vi "test_NEO480HTA get all data.vi"(8 "Error In":errorcluster) -> (0 "Error Out":errorcluster)   [LabVIEW 2023]
uses:
  Real All CFG/Read All CFG.lvclass
  Virt Instr Host/Virt Instr Host.lvclass
  Measure and Stimulus Subsystems/Measure and Stimulus Subsystems.lvclass
panel:
  out "i":i32
  out "Absolute Humidity":dbl format="%#_g g m^-3"
  out "Pressure":dbl format="%#_g mbar"
  out "Dew Point":dbl format="%#_g °C"
  out "Temperature":dbl format="%#_g °C"
  in  "Stop":bool
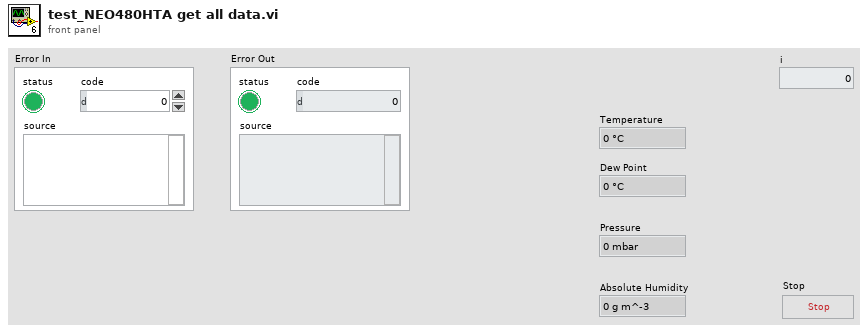
[diagram p1: front panel]
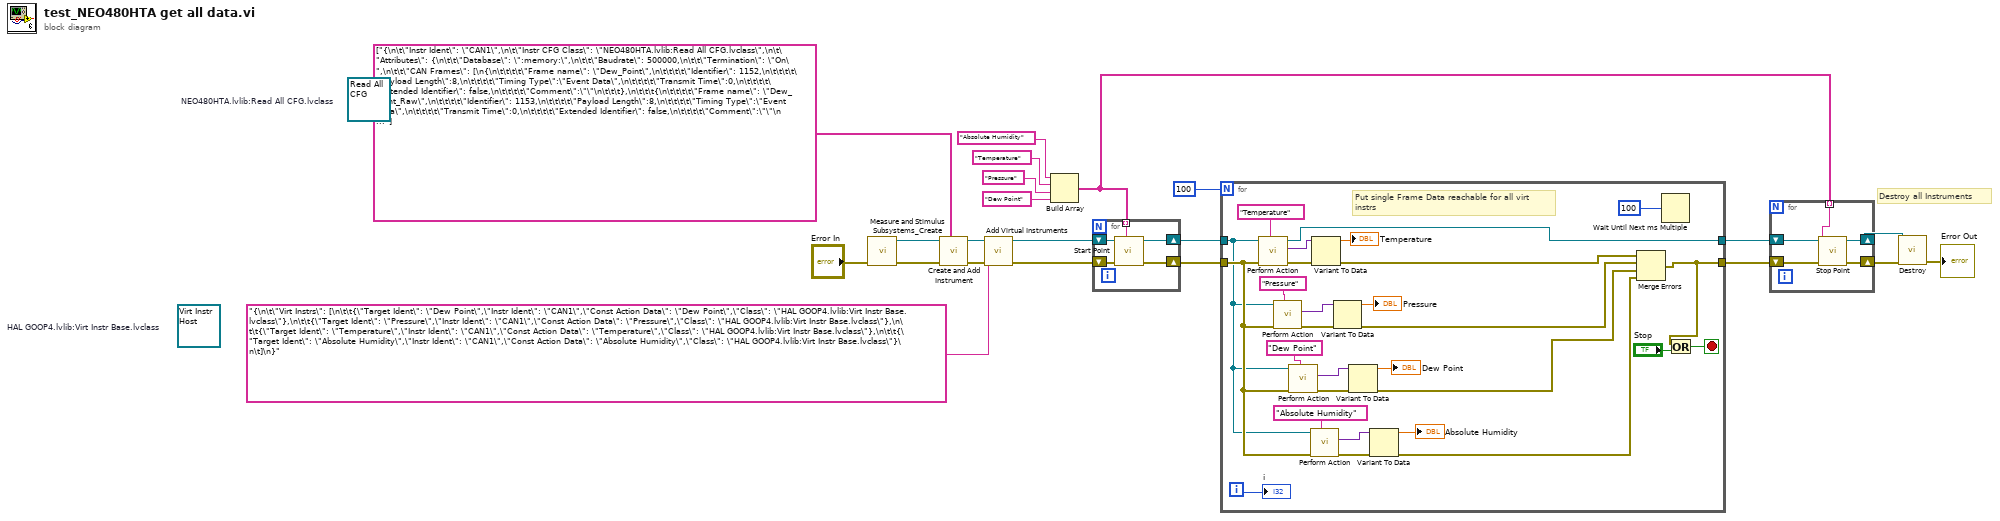
[diagram p0: block diagram]
diagram:
  (unwired) refnum<class "Virt Instr Host.lvclass"> refnum  # HAL GOOP4.lvlib:Virt Instr Base.lvclass
  (unwired) refnum<class "Read All CFG.lvclass"> refnum  # NEO480HTA.lvlib:Read All CFG.lvclass
  # "Destroy all Instruments"
  n1 = call "Measure and Stimulus Subsystems_Create.vi"("Error In"="Error In") -> ("Error Out"=w21:errorcluster, "reference out"=w22:refnum<class "Measure and Stimulus Subsystems.lvclass">)  [unwired: 9 in]
  n2 = call "Create and Add Instrument.vi"("Physical Intr Configs"=string[] ["{\n\t\"Instr Ident\": \"CAN1\",\n\t\"Instr CFG Class\": \"NEO480HTA.lvlib:Read All CFG.lvclass\",\n\t\"Attributes\": {\n\t\t\"Database\": \":memory:\",\n\t\t\"Baudrate\": 500000,\n\t\t\"Termination\": \"On\",\n\t\t\"CAN Frames\": [\n{\n\t\t\t\t\"Frame name\": \"Dew_Point\",\n\t\t\t\t\"Identifier\": 1152,\n\t\t\t\t\"Payload Length\":8,\n\t\t\t\t\"Timing Type\":\"Event Data\",\n\t\t\t\t\"Transmit Time\":0,\n\t\t\t\t\"Extended Identifier\": false,\n\t\t\t\t\"Comment\":\"\"\n\t\t\t},\n\t\t\t{\n\t\t\t\t\"Frame name\": \"Dew_Point_Raw\",\n\t\t\t\t\"Identifier\": 1153,\n\t\t\t\t\"Payload Length\":8,\n\t\t\t\t\"Timing Type\":\"Event Data\",\n\t\t\t\t\"Transmit Time\":0,\n\t\t\t\t\"Extended Identifier\": false,\n\t\t\t\t\"Comment\":\"\"\n                      }\n],\n\t\t\"Acquire\": {\n\t\t\t\"Type\": \"Read Frame\"\n\t\t}\n\t}\n}"], "Error In"=w21, "reference in"=w22) -> ("Error Out"=w18:errorcluster, "reference out"=w13:refnum<class "Measure and Stimulus Subsystems.lvclass">)  [unwired: 7 in]
  n3 = call-dynamic "Add Virtual Instruments.vi"("error in"=w18, "<JSON CFG>"="{\n\t\"Virt Instrs\": [\n\t\t{\"Target Ident\": \"Dew Point\",\"Instr Ident\": \"CAN1\",\"Const Action Data\": \"Dew Point\",\"Class\": \"HAL GOOP4.lvlib:Virt Instr Base.lvclass\"},\n\t\t{\"Target Ident\": \"Pressure\",\"Instr Ident\": \"CAN1\",\"Const Action Data\": \"Pressure\",\"Class\": \"HAL GOOP4.lvlib:Virt Instr Base.lvclass\"},\n\t\t{\"Target Ident\": \"Temperature\",\"Instr Ident\": \"CAN1\",\"Const Action Data\": \"Temperature\",\"Class\": \"HAL GOOP4.lvlib:Virt Instr Base.lvclass\"},\n\t\t{\"Target Ident\": \"Absolute Humidity\",\"Instr Ident\": \"CAN1\",\"Const Action Data\": \"Absolute Humidity\",\"Class\": \"HAL GOOP4.lvlib:Virt Instr Base.lvclass\"}\n\t]\n}", "Host Measure and Stimulus Subsystems in"=w13) -> ("error out"=w14:errorcluster, "Host Measure and Stimulus Subsystems out"=w12:refnum<class "Measure and Stimulus Subsystems.lvclass">)  [unwired: 7 in]
  n4 = Build Array("Absolute Humidity" ("Target Ident"), "Temperature" ("Target Ident"), "Pressure" ("Target Ident"), "Dew Point" ("Target Ident")) -> (w1:string[])
  n5 = for {
    shift-right: [w27] -> w16
    shift-left: w14 -> [w26]
    shift-right: [w24] -> w10
    shift-left: w12 -> [w25]
    tunnel: w1 -> [w23] mode=indexing
    n6 = call-dynamic "Start Point.vi"("Position Ident"=w23, "error in"=w26, "Measure and Stimulus Subsystems in"=w25) -> ("error out"=w27:errorcluster, "Measure and Stimulus Subsystems out"=w24:refnum<class "Measure and Stimulus Subsystems.lvclass">)  [unwired: 7 in]
  }
  n7 = for {
    N: 100 -> [_]
    tunnel: w16 -> [w38]
    tunnel: w10 -> [w37]
    tunnel: [w35] -> w2
    tunnel: [w32] -> w3
    i -> [w28]
    stop <- w55 stop-if-true
    # "Put single Frame Data reachable for all virt\ninstrs"
    n8 = call-dynamic "Perform Action.vi"("Point Ident"="Temperature" ("Target Identifier"), "error in"=w38, "Host Measure and Stimulus Subsystems in"=w37) -> ("error out"=w49:errorcluster, "Output"=w48:variant, "Host Measure and Stimulus Subsystems out"=w35:refnum<class "Measure and Stimulus Subsystems.lvclass">)  [unwired: 6 in]
    n9 = call-dynamic "Perform Action.vi"("Point Ident"="Pressure" ("Target Identifier"), "error in"=w38, "Host Measure and Stimulus Subsystems in"=w37) -> ("error out"=w53:errorcluster, "Output"=w51:variant)  [unwired: 6 in, 1 out]
    n10 = call-dynamic "Perform Action.vi"("Point Ident"="Dew Point" ("Target Identifier"), "error in"=w38, "Host Measure and Stimulus Subsystems in"=w37) -> ("error out"=w45:errorcluster, "Output"=w43:variant)  [unwired: 6 in, 1 out]
    n11 = call-dynamic "Perform Action.vi"("Point Ident"="Absolute Humidity" ("Target Identifier"), "error in"=w38, "Host Measure and Stimulus Subsystems in"=w37) -> ("error out"=w39:errorcluster, "Output"=w41:variant)  [unwired: 6 in, 1 out]
    n12 = Variant To Data(error in=w49, Variant=w48) -> (data=→"Temperature":dbl, error out=w34:errorcluster)  [unwired: 1 in]
    n13 = Variant To Data(error in=w53, Variant=w51) -> (data=→"Pressure":dbl, error out=w33:errorcluster)  [unwired: 1 in]
    n14 = Variant To Data(error in=w45, Variant=w43) -> (data=→"Dew Point":dbl, error out=w31:errorcluster)  [unwired: 1 in]
    n15 = Variant To Data(error in=w39, Variant=w41) -> (data=→"Absolute Humidity":dbl, error out=w30:errorcluster)  [unwired: 1 in]
    n16 = Merge Errors(w34, w33, w31, w30) -> (w32:errorcluster)
    n17 = Wait Until Next ms Multiple(millisecond multiple=u32 100) -> ()  [unwired: 1 out]
    n18 = Or(x=w32, y="Stop") -> (x .or. y?=w55:bool)
    "i" <- w28
  }
  n19 = for {
    shift-right: [w59] -> w4
    shift-left: w3 -> [w58]
    shift-right: [w60] -> w5
    shift-left: w2 -> [w57]
    tunnel: w1 -> [w56] mode=indexing
    n20 = call-dynamic "Stop Point.vi"("error in"=w58, "Point Ident"=w56, "Host Measure and Stimulus Subsystems in"=w57) -> ("error out"=w59:errorcluster, "Host Measure and Stimulus Subsystems out"=w60:refnum<class "Measure and Stimulus Subsystems.lvclass">)  [unwired: 7 in]
  }
  n21 = call-dynamic "Destroy.vi"("Error In"=w4, "reference in"=w5) -> ("Error Out"=→"Error Out":errorcluster)  [unwired: 8 in, 1 out]
